vi "Constructor.vi"(8 "error in":errorcluster, 9 "AlicatSetup":T1, 10 "SP":sgl, 11 "Alicat Controller in":refnum<class "Alicat Controller.lvclass">) -> (0 "error out":errorcluster, 3 "Alicat Controller out":refnum<class "Alicat Controller.lvclass">)   [LabVIEW 2015, in "Alicat.lvlib" / "Alicat Controller.lvclass"]
uses:
  Alicat Controller.lvclass
  Controls/CtlSetup.ctl
  Controls/Gas.ctl
  Alicat Controller.lvclass/Alicat Controller.ctl
  Alicat.lvclass
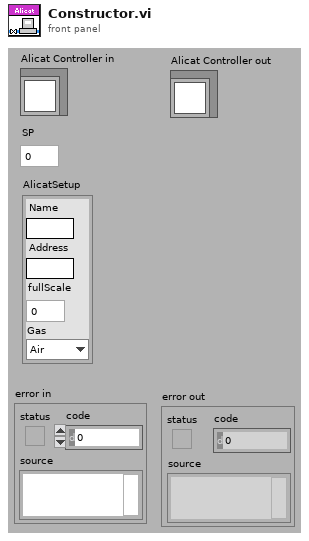
[diagram p1: front panel]
types:
  T1 = typedef "Alicat.lvlib/Alicat.lvclass/CtlSetup.ctl" = cluster{"Name":string, "Address":string, "fullScale":dbl, "Gas":T2}
  T2 = typedef "Alicat.lvlib/Alicat.lvclass/Gas.ctl" = enum16{"Air", "Ar", "CH4", "CO", "CO2", "C2H6", "H2", "He", "N2", "NO", "Ne", "O2", "C3H8", "n-C4H10", "C2H2", "C2H4", "i-C2H10", "Kr", "Xe"}
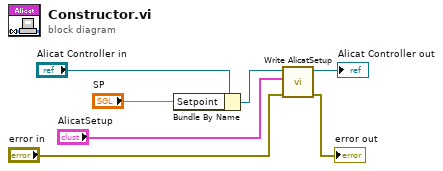
[diagram p0: block diagram]
diagram:
  n1 = Bundle By Name(cluster="Alicat Controller in", "Setpoint"="SP") -> (w1:refnum<class "Alicat Controller.lvclass">)
  n2 = call "Write AlicatSetup.vi"("error in"="error in", "AlicatSetup"="AlicatSetup", "Alicat in"=w1) -> ("error out"=→"error out":errorcluster, "Alicat out"=→"Alicat Controller out":refnum<class "Alicat Controller.lvclass">)  [unwired: 7 in]
